vi "ASK_AddCRC.vi"(8 "error in (no error)":errorcluster caption="错误输入（无错误）", 9 "crc_num":i32, 10 "input_data":dbl[](array[numeric]) format="%#_13g", 11 "PathIn":path) -> (0 "error out":errorcluster caption="错误输出", 2 "output_data":dbl[](array[numeric]), 3 "PathOut":path)   [LabVIEW 2015]
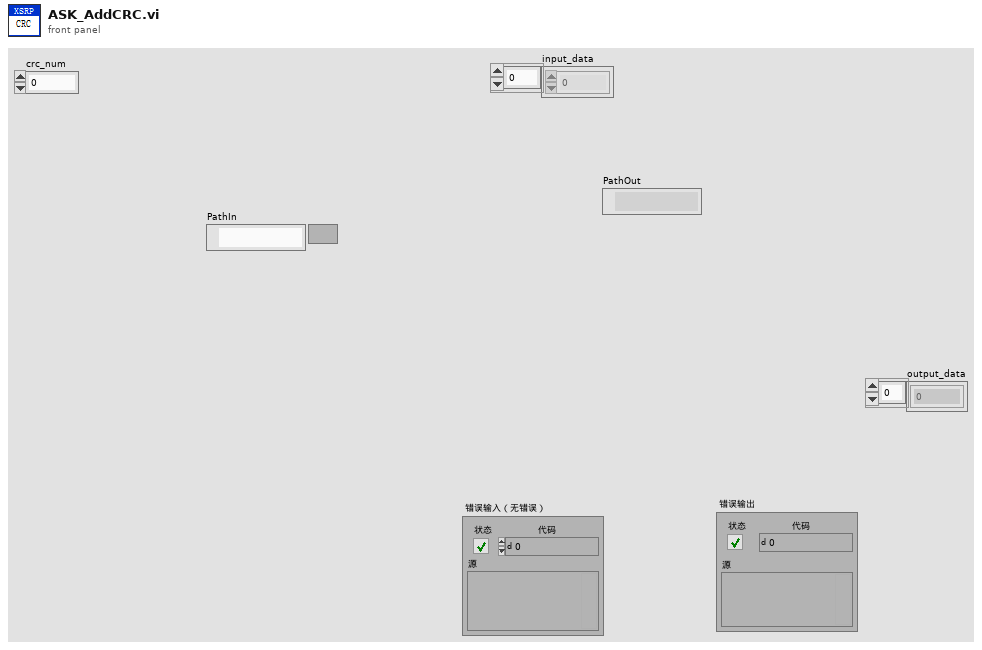
[diagram p1: front panel]
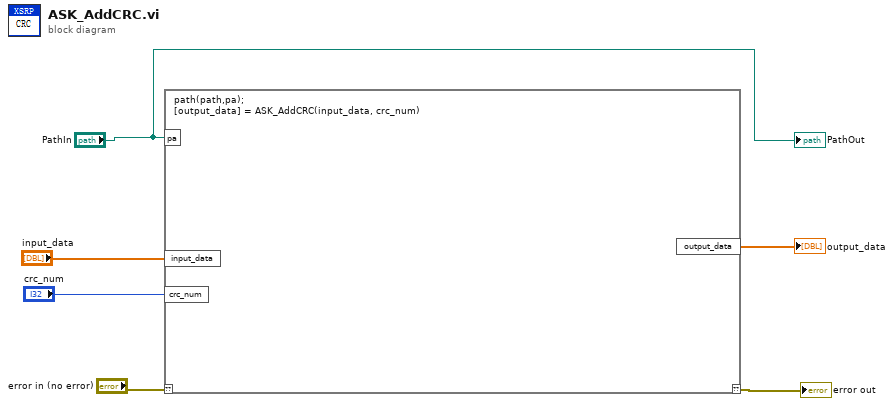
[diagram p0: block diagram]
diagram:
  n1 = script code="path(path,pa);\n[output_data] = ASK_AddCRC(input_data, crc_num)"("??"="error in (no error)", "pa"="PathIn", "input_data"="input_data", "crc_num"="crc_num") -> ("??"=→"error out":errorcluster, "output_data"=→"output_data":dbl[])
  "PathOut" <- "PathIn"
